vi "WSVCAP SHL FPGA LL Procedure I2C - Send Start or Stop Sequence.vi"(0 "Procedure Step":T1, 1 "Wait Ticks Remaining":u32, 5 "I2C Wait Ticks":u32, 11 "error in (no error)":errorcluster, 12 "Type (T:Start; F:Stop)":bool, 13 "Socket Mask":u64) -> (3 "Wait Ticks Remaining Out":u32, 4 "Procedure Step Out":T1, 8 "Finished":bool, 15 "error out":errorcluster)   [LabVIEW 2012]
uses:
  Type Defs/WSVCAP SHL Procedure Step Enum.ctl
  Type Defs/WSVCAP SHL I2C Write Line Enum.ctl
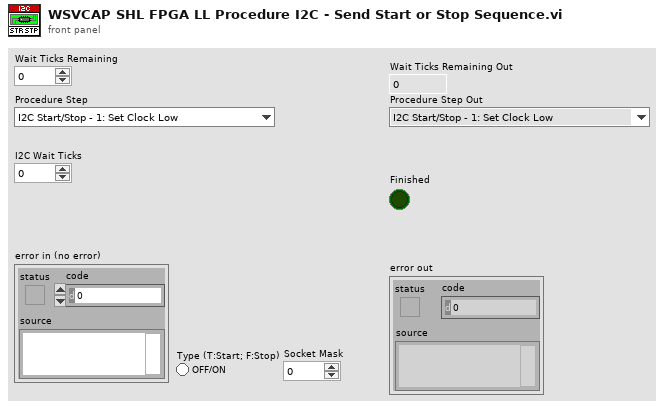
[diagram p1: front panel]
types:
  T1 = typedef "WSVCAP SHL Procedure Step Enum.ctl" = enum16{"I2C Start/Stop - 1: Set Clock Low", "I2C Start/Stop - 2: Wait", "I2C Start/Stop - 3: Set Data I", "I2C Start/Stop - 4: Wait", "I2C Start/Stop - 5: Set Clock High", "I2C Start/Stop - 6: Wait", "I2C Start/Stop - 7: Set Data II", "I2C Start/Stop - 8: Wait", "I2C Start/Stop - 9: Set Clock Low", "I2C Start/Stop - 10: Wait", "I2C Read ACK - 1: Set Clock High", "I2C Read ACK - 2: Wait", "I2C Read ACK - 3: Read ACK Bit", "I2C Read ACK - 4: Wait", "I2C Read ACK - 5: Set Clock Low", "I2C Read ACK - 6: Wait", "I2C Write ACK - 1: Write ACK Bit", "I2C Write ACK - 2: Wait", "I2C Write ACK - 3: Set Clock High", "I2C Write ACK - 4: Wait", "I2C Write ACK - 5: Set Clock Low", "I2C Write ACK - 6: Wait", "I2C Write ACK - 7: Set Data Low", "I2C Send Add - 1: Reset Bits Remaining", "I2C Send Add - 2: Set Data Bit", "I2C Send Add - 3: Wait", "I2C Send Add - 4: Set Clock High", "I2C Send Add - 5: Wait", "I2C Send Add - 6: Set Clock Low", "I2C Send Add - 7: Wait", "I2C Send Add - 8: Check Bits Remaining", "I2C Send Data - 1: Reset Bits Remaining", "I2C Send Data - 2: Load Write Bit from FIFO", "I2C Send Data - 3: Set Data Bit", "I2C Send Data - 4: Wait", "I2C Send Data - 5: Set Clock High", "I2C Send Data - 6: Wait", "I2C Send Data - 7: Set Clock Low", "I2C Send Data - 8: Wait", "I2C Send Data - 9: Check Bits Remaining", "I2C Receive Data - 1: Reset Bits Remaining", "I2C Receive Data - 2: Wait", "I2C Receive Data - 3: Set Clock High", "I2C Receive Data - 4: Wait", "I2C Receive Data - 5: Read Data Bit", "I2C Receive Data - 6: Wait", "I2C Receive Data - 7: Set Clock Low", "I2C Receive Data - 8: Wait", "I2C Receive Data - 9: Check Bits Remaining", "SPI Clear Lines - 1:Clear", "SPI Send/Receive - 1: Load SDA - Clock Low", "SPI Send/Receive - 2: Wait", "SPI Send/Receive - 3: Load DATO - Clock High", "SPI Send/Receive - 4: Wait", "SPI Wait CMD Delay - 1:Wait", "RFFE Send SSC - 1:Set Low", "RFFE Send SSC - 2:Wait", "RFFE Send SSC - 3:Set SDA High", "RFFE Send SSC - 4:Wait", "RFFE Send SSC - 5:Set SDA Low", "RFFE Send SSC - 6:Wait", "RFFE Send Data - 1:Set SCL High", "RFFE Send Data - 2:Wait", "RFFE Send Data - 3:Set SCL Low", "RFFE Send Data - 4:Wait", "RFFE Send Data - 5:Set SCL High (P)", "RFFE Send Data - 6:Wait", "RFFE Send Data - 7:Set SCL Low (P)", "RFFE Send Data - 8:Wait", "RFFE Send Data - 9:Set SCL High (BP)", "RFFE Send Data - 10:Wait", "RFFE Send Data - 11:Set SCL Low (BP)", "RFFE Send Data - 12:Wait", "RFFE Receive Data - 1:Set SCL High", "RFFE Receive Data - 2:Wait", "RFFE Receive Data - 3:Set SCL Low", "RFFE Receive Data - 4:Wait", "RFFE Receive Data - 5:Set SCL High (BP)", "RFFE Receive Data - 6:Wait", "RFFE Receive Data - 7:Set SCL Low (BP)", "RFFE Receive Data - 8:Wait", "RFFE Wait CMD Delay - 1:Wait", "RFFE Clear Lines - 1:Clear"}
  T2 = typedef "WSVCAP SHL I2C Write Line Enum.ctl" = enum16{"I2C SCL", "I2C SDA"}
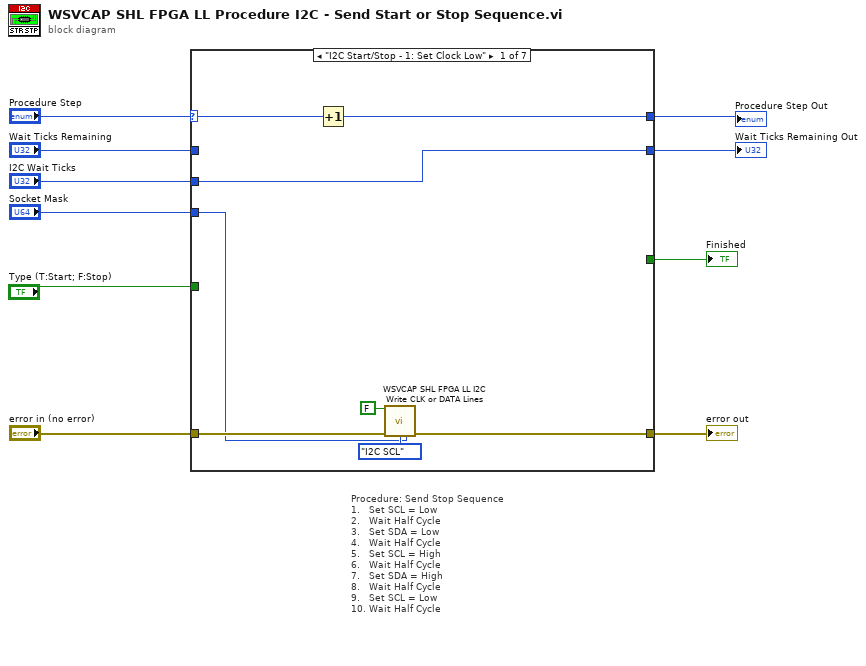
[diagram p0: block diagram]
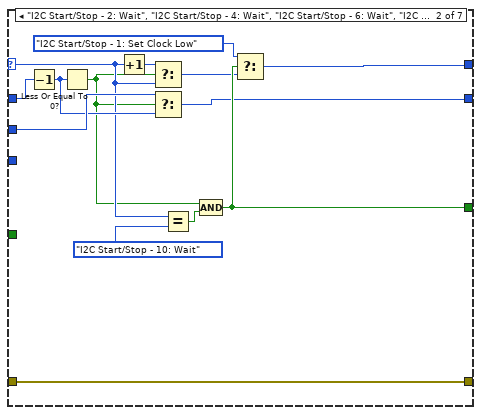
[diagram p2: hidden frame]
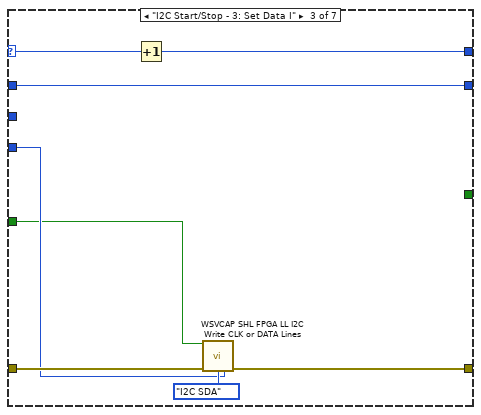
[diagram p3: hidden frame]
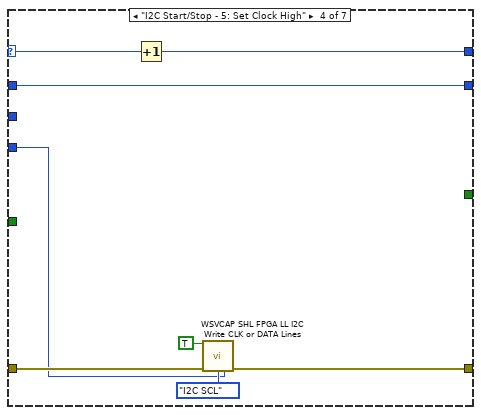
[diagram p4: hidden frame]
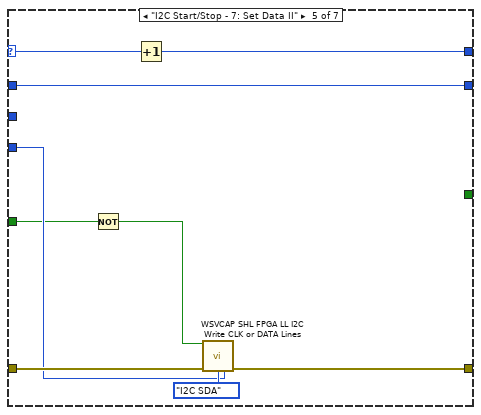
[diagram p5: hidden frame]
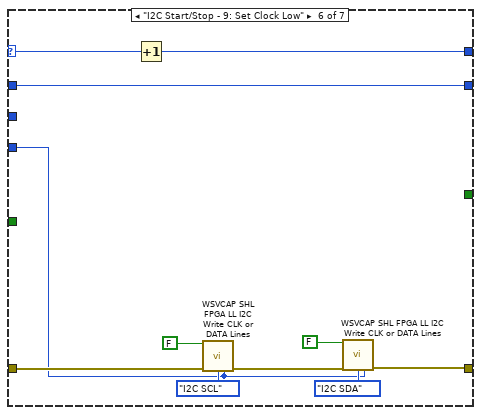
[diagram p6: hidden frame]
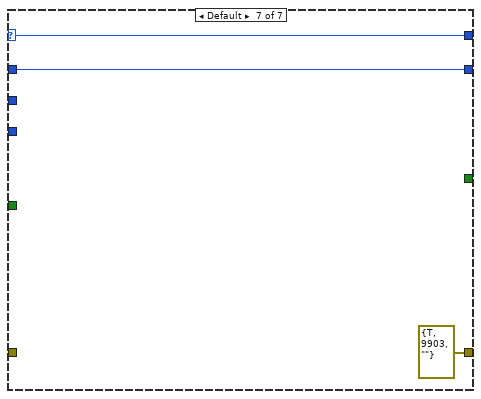
[diagram p7: hidden frame]
diagram:
  # "Procedure: Send Stop Sequence\n1.   Set SCL = Low\n2.   Wait Half Cycle\n3.   Set SDA = Low\n4.   Wait Half Cycle\n5.   Set SCL = High\n6.   Wait Half Cycle\n7.   Set SDA = High\n8.   Wait Half Cycle\n9.   Set SCL = Low\n10. Wait Half Cycle"
  n1 = case shown="\"I2C Start/Stop - 1: Set Clock Low\"" "Procedure Step" {
    selector: "Procedure Step" -> [w14 w27 w37 w44 w54 w65 w70]
    tunnel: [w16 w30 w38 w46 w55 w61 errorcluster {"status"=TRUE, "code"=9903, "source"=""} ("error out")] -> w9
    tunnel: "error in (no error)" -> [w17 w30 w39 w47 w56 w67 _]
    tunnel: "Wait Ticks Remaining" -> [_ w32 w33 w41 w49 w58 w69]
    tunnel: "I2C Wait Ticks" -> [w11 w29 _ _ _ _ _]
    tunnel: [_ w24 _ _ _ _ _] -> w8
    tunnel: "Socket Mask" -> [w13 _ w36 w43 w52 w60 _]
    tunnel: "Type (T:Start; F:Stop)" -> [_ _ w35 _ w51 _ _]
    tunnel: [w12 w20 w34 w42 w50 w59 w70] -> w2
    tunnel: [w11 w19 w33 w41 w49 w58 w69] -> w1
    frame "I2C Start/Stop - 1: Set Clock Low" {
      n2 = Increment(x=w14) -> (x+1=w12:T1)
      n3 = call "WSVCAP SHL FPGA LL I2C Write CLK or DATA Lines.vi"("Bit In"=FALSE, "error in (no error)"=w17, "Line"=WSVCAP_SHL_I2C_Write_Line_Enum."I2C SCL", "Socket Mask"=w13) -> ("error out"=w16:errorcluster)  [unwired: 11 in]
    }
    frame "I2C Start/Stop - 2: Wait", "I2C Start/Stop - 4: Wait", "I2C Start/Stop - 6: Wait", "I2C Start/Stop - 8: Wait", "I2C Start/Stop - 10: Wait" {
      n4 = Decrement(x=w32) -> (x-1=w28:u32)
      n5 = Less Or Equal To 0?(x=w28) -> (x <= 0?=w26:bool)
      n6 = Increment(x=w27) -> (x+1=w31:T1)
      n7 = Select(t=w31, s=w26, f=w27) -> (s? t:f=w23:T1)
      n8 = Select(t=w29, s=w26, f=w28) -> (s? t:f=w19:u32)
      n9 = Equal?(x=w27, y=WSVCAP_SHL_Procedure_Step_Enum."I2C Start/Stop - 10: Wait" ("Procedure Step")) -> (x = y?=w25:bool)
      n10 = Compound Arithmetic op=AND(w26, w25) -> (w24:bool)
      n11 = Select(t=WSVCAP_SHL_Procedure_Step_Enum."I2C Start/Stop - 1: Set Clock Low" ("Procedure Step"), s=w24, f=w23) -> (s? t:f=w20:T1)
    }
    frame "I2C Start/Stop - 3: Set Data I" {
      n12 = Increment(x=w37) -> (x+1=w34:T1)
      n13 = call "WSVCAP SHL FPGA LL I2C Write CLK or DATA Lines.vi"("Bit In"=w35, "error in (no error)"=w39, "Line"=WSVCAP_SHL_I2C_Write_Line_Enum."I2C SDA", "Socket Mask"=w36) -> ("error out"=w38:errorcluster)  [unwired: 11 in]
    }
    frame "I2C Start/Stop - 5: Set Clock High" {
      n14 = Increment(x=w44) -> (x+1=w42:T1)
      n15 = call "WSVCAP SHL FPGA LL I2C Write CLK or DATA Lines.vi"("Bit In"=TRUE, "error in (no error)"=w47, "Line"=WSVCAP_SHL_I2C_Write_Line_Enum."I2C SCL", "Socket Mask"=w43) -> ("error out"=w46:errorcluster)  [unwired: 11 in]
    }
    frame "I2C Start/Stop - 7: Set Data II" {
      n16 = Not(x=w51) -> (.not. x?=w53:bool)
      n17 = Increment(x=w54) -> (x+1=w50:T1)
      n18 = call "WSVCAP SHL FPGA LL I2C Write CLK or DATA Lines.vi"("Bit In"=w53, "error in (no error)"=w56, "Line"=WSVCAP_SHL_I2C_Write_Line_Enum."I2C SDA", "Socket Mask"=w52) -> ("error out"=w55:errorcluster)  [unwired: 11 in]
    }
    frame "I2C Start/Stop - 9: Set Clock Low" {
      n19 = Increment(x=w65) -> (x+1=w59:T1)
      n20 = call "WSVCAP SHL FPGA LL I2C Write CLK or DATA Lines.vi"("Bit In"=FALSE, "error in (no error)"=w67, "Line"=WSVCAP_SHL_I2C_Write_Line_Enum."I2C SCL", "Socket Mask"=w60) -> ("error out"=w62:errorcluster)  [unwired: 11 in]
      n21 = call "WSVCAP SHL FPGA LL I2C Write CLK or DATA Lines.vi"("Bit In"=FALSE, "error in (no error)"=w62, "Line"=WSVCAP_SHL_I2C_Write_Line_Enum."I2C SDA", "Socket Mask"=w60) -> ("error out"=w61:errorcluster)  [unwired: 11 in]
    }
    frame Default {
    }
  }
  "error out" <- w9
  "Finished" <- w8
  "Wait Ticks Remaining Out" <- w1
  "Procedure Step Out" <- w2
